vi "multiple_sources.vi"() -> ()   [LabVIEW 2021]
panel:
  out "output":dbl
  out "input 2":dbl
  in  "input 1":dbl
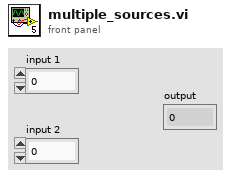
[diagram p1: front panel]
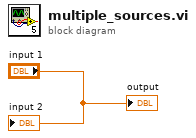
[diagram p0: block diagram]
diagram:
  "input 2" <- "input 1"
  "output" <- "input 1"
